vi "FTW-TestExecutive-Core_Stop.vi"(0 "FTW-Scripter-Core In":refnum<class "FTW-TestExecutive-Core.lvclass">, 11 "error in":errorcluster) -> (4 "FTW-Scripter-Core Out":refnum<class "FTW-TestExecutive-Core.lvclass">, 15 "error out":errorcluster)   [LabVIEW 2015, in "FTW-TestExecutive-Core.lvclass"]
uses:
  FTW-TestExecutive-Core.lvclass
  FTW-TestExecutive-Core.lvclass/FTW-TestExecutive-Core.ctl
  FTW-TestExecutive-Step-State.ctl
  FTW-TestExecutive-Core_State.ctl
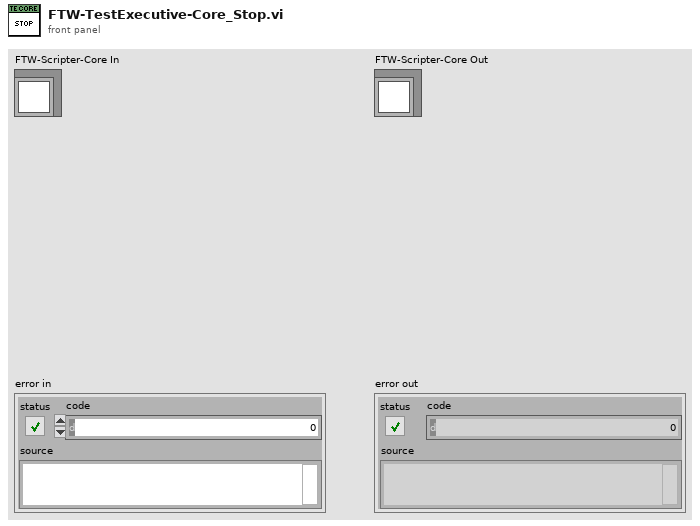
[diagram p1: front panel]
types:
  T1 = typedef "FTW-TestExecutive-Core.lvclass/FTW-TestExecutive-Core_State.ctl" = enum8{"Unloaded", "Loaded", "Executing", "Paused"}
  T2 = typedef "FTW-TestExecutive-Step-State.ctl" = enum8{"None", "Failed", "Passed", "Timed out", "Aborted"}
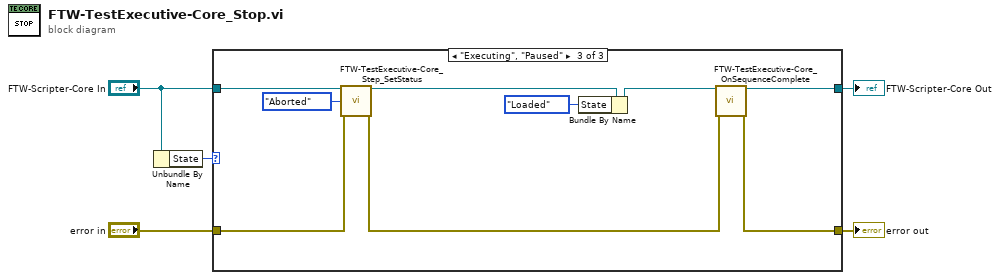
[diagram p0: block diagram]
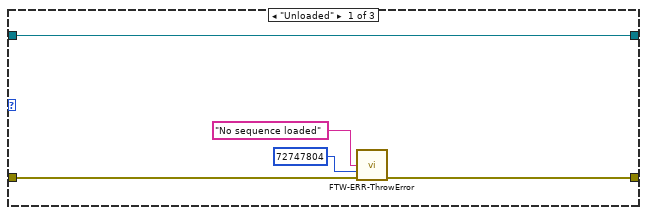
[diagram p2: hidden frame]
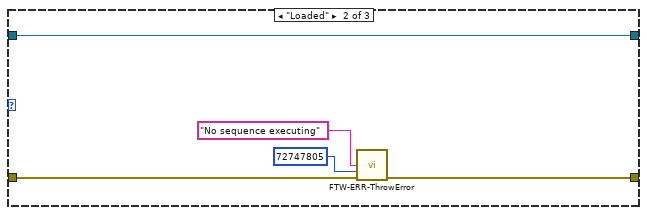
[diagram p3: hidden frame]
diagram:
  n1 = Unbundle By Name("FTW-Scripter-Core In") -> ("State"=w3:T1)
  n2 = case shown="\"Executing\", \"Paused\"" w3 {
    tunnel: [w10 w15 w18] -> w5
    tunnel: "FTW-Scripter-Core In" -> [w10 w15 w24]
    tunnel: [w8 w13 w17] -> w2
    tunnel: "error in" -> [w9 w14 w21]
    frame "Unloaded" {
      n3 = call "FTW-ERR-ThrowError.vi"("Error Message"="No sequence loaded", "Error Code"=72747804, "error in"=w9) -> ("error out"=w8:errorcluster)  [unwired: 12 in]
    }
    frame "Loaded" {
      n4 = call "FTW-ERR-ThrowError.vi"("Error Message"="No sequence executing", "Error Code"=72747805, "error in"=w14) -> ("error out"=w13:errorcluster)  [unwired: 12 in]
    }
    frame "Executing", "Paused" {
      n5 = call "FTW-TestExecutive-Core_Step_SetStatus.vi"("FTW-Scripter-Core In"=w24, "State"=FTW-TestExecutive-Step-State."Aborted", "error in"=w21) -> ("FTW-Scripter-Core Out"=w23:refnum<class "FTW-TestExecutive-Core.lvclass">, "error out"=w16:errorcluster)  [unwired: 11 in]
      n6 = Bundle By Name(cluster=w23, "State"=FTW-TestExecutive-Core_State."Loaded") -> (w20:refnum<class "FTW-TestExecutive-Core.lvclass">)
      n7 = call "FTW-TestExecutive-Core_OnSequenceComplete.vi"("FTW-Scripter-Core In"=w20, "error in"=w16) -> ("FTW-Scripter-Core Out"=w18:refnum<class "FTW-TestExecutive-Core.lvclass">, "error out"=w17:errorcluster)  [unwired: 12 in]
    }
  }
  "FTW-Scripter-Core Out" <- w5
  "error out" <- w2
